vi "TDC_resetHbtCorrelations.vi"(8 "Error In":errorcluster) -> (0 "Error Out":errorcluster)   [LabVIEW 2011]
uses:
  tdcbase.dll
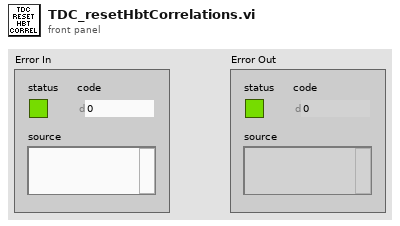
[diagram p1: front panel]
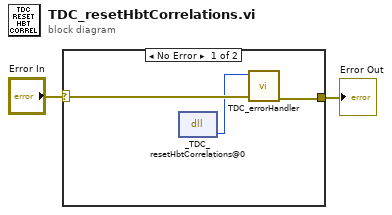
[diagram p0: block diagram]
diagram:
  n1 = case shown="No Error" "Error In" {
    selector: "Error In" -> [w5 w6]
    tunnel: [w4 w6] -> w1
    frame No Error {
      n2 = dll-call lib="X:/tdcbase.dll" fn="_TDC_resetHbtCorrelations@0"() -> ("return type"=w3:i32)  [unwired: 3 in, 2 out]
      n3 = call "TDC_errorHandler.vi"("Error In"=w5, "TDC Return Code"=w3) -> ("Error Out"=w4:errorcluster)  [unwired: 9 in]
    }
    frame Error {
    }
  }
  "Error Out" <- w1
